vi "Error 5007 - Unrecognized Error While Processing ProtoBuf Message.vi"() -> (0 "error out":errorcluster)   [LabVIEW 2020]
doc: "Error 5007 - Unrecognized Error While Processing ProtoBuf Message"
uses:
  <vilib>/Utility/error.llb/Error Cluster From Error Code.vi
  <vilib>/ErrorRing/Error Ring.xnode
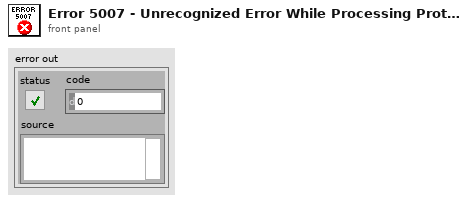
[diagram p1: front panel]
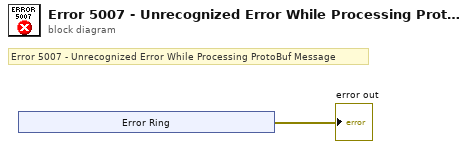
[diagram p0: block diagram]
diagram:
  # "Error 5007 - Unrecognized Error While Processing ProtoBuf Message"
  n1 = xnode "Error Ring"() -> ("error out"=→"error out":errorcluster)
